vi "HAL camera program for acquisition.vi"(2 "error in":errorcluster, 3 "Camera Parameters (important)":T1={"Exposure Time (sec)"=0.0, "EM CCD Gain"=0, "Readout Settings"={"Acquisition Mode"=enum."(do not use)", "Pixel Rate"=enum."EM CCD 30 Mhz 16 bits", "High Capacity?"=FALSE, "V Shift Speed (us/row)"=enum."4.33", "V Shift Amplitude"=enum."normal", "Preamp Gain"=enum."1", "Trigger Mode"=0, "Baseline offset"=0, "Baseline clamp"=FALSE}, "Image Size"={"H Bin"=0, "V Bin"=0, "Left"=0, "Top"=0, "Right"=0, "Bottom"=0}} {"Readout Settings"."Baseline offset" min=-1000 max=1000 step=100; "Readout Settings"."Trigger Mode" items=["Internal", "External"]; "EM CCD Gain" scale=1.0..300.0; "Exposure Time (sec)" scale=0.001..10.0 scale format="%#_1g"}) -> (0 "error out":errorcluster, 1 "Actual Exposure Time (sec)":sgl)   [LabVIEW 2015]
uses:
  ixon ultra1024/HAL camera parameters important.ctt
  ixon ultra1024/ixon readout settings.ctl
  ixon ultra1024/andor acquisition mode.ctl
  Camera/camera globals.vi
panel:
  # "Camera: Andor iXon Ultra"
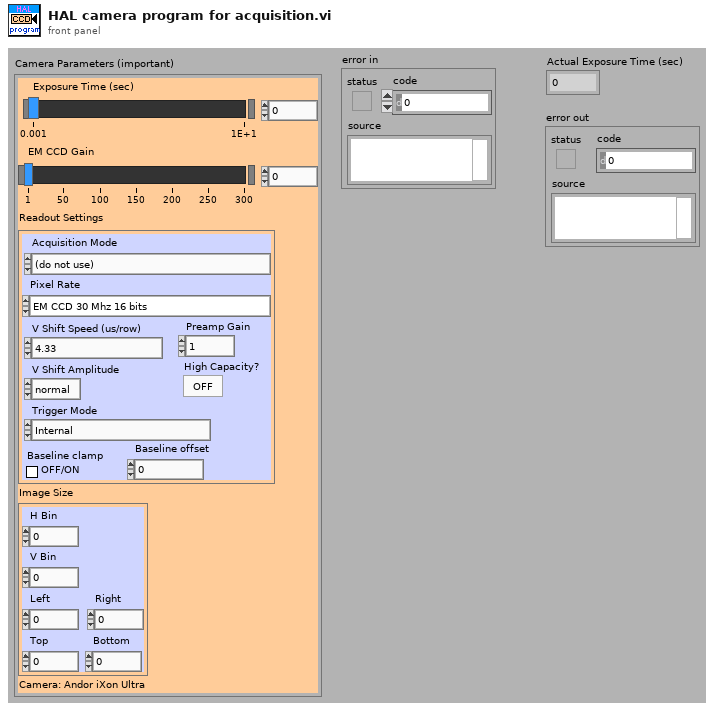
[diagram p1: front panel]
types:
  T1 = typedef "HAL camera parameters important.ctt" = cluster{"Exposure Time (sec)":sgl, "EM CCD Gain":u16, "Readout Settings":T2, "Image Size":cluster{"H Bin":i32, "V Bin":i32, "Left":i32, "Top":i32, "Right":i32, "Bottom":i32}}
  T2 = typedef "ixon readout settings.ctl" = cluster{"Acquisition Mode":T3, "Pixel Rate":enum16{"EM CCD 30 Mhz 16 bits", "EM CCD 20 Mhz 16 bits", "EM CCD 10 Mhz 16 bits", "EM CCD 1 Mhz 16 bits", "Standard CCD 1 Mhz 16 bits", "Standard CCD 0.1 Mhz 16 bits"}, "High Capacity?":bool, "V Shift Speed (us/row)":enum16{"0.6 (not reccommended)", "1.13  (not reccommended)", "2.2  (not reccommended)", "4.33"}, "V Shift Amplitude":enum16{"normal", "+1", "+2", "+3", "+4"}, "Preamp Gain":enum16{"1", "2", "3"}, "Trigger Mode":u32, "Baseline offset":i16, "Baseline clamp":bool}
  T3 = typedef "andor acquisition mode.ctl" = enum16{"(do not use)", "Single Scan", "Accumulate", "Kinetics", "Fast Kinetics", "Kinetics Run till Abort", "Frame Transfer", "Frame Transfer Run till Abort", "(do not use) ", "Time Delayed Integration"}
  T4 = cluster{"H Bin":i32, "V Bin":i32, "Left":i32, "Top":i32, "Right":i32, "Bottom":i32}
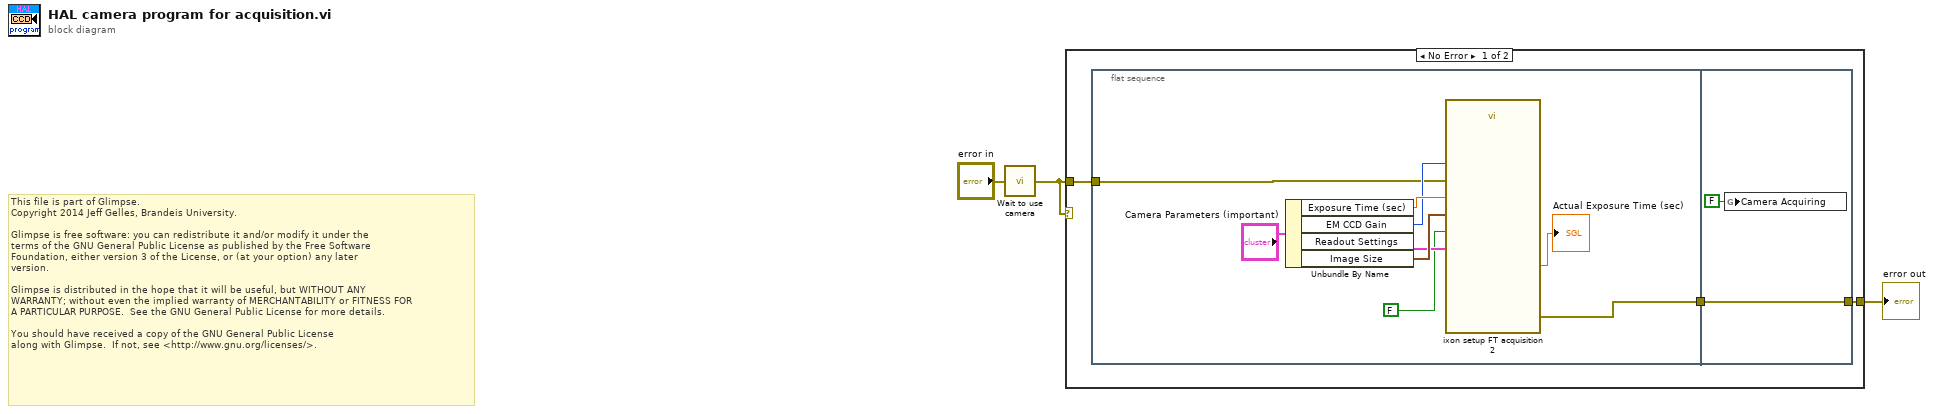
[diagram p0: block diagram]
diagram:
  # "This file is part of Glimpse. \nCopyright 2014 Jeff Gelles, Brandeis University.    \n\nGlimpse is free software: you can redistribute it and/or modify it under the \nterms of the GNU General Public License as published by the Free Software \nFoundation, either version 3 of the License, or (at your option) any later \nversion.\n\nGlimpse is distributed in the hope that it will be useful, but WITHOUT ANY \nWARRANTY; without even the implied warranty of MERCHANTABILITY or FITNESS FOR \nA PARTICULAR PURPOSE.  See the GNU General Public License for more details.\n\nYou should have received a copy of the GNU General Public License\nalong with Glimpse.  If not, see <http://www.gnu.org/licenses/>."
  n1 = call "Wait to use camera.vi"("error in"="error in") -> ("error out"=w1:errorcluster)
  n2 = case shown="No Error" w1 {
    tunnel: [w6 w18] -> w3
    tunnel: w1 -> [w5 w18]
    frame No Error {
      n3 = flat-sequence {
        tunnel: w5 -> [w7]
        tunnel: [w15] -> w4
        tunnel: [w17] -> w6
        tunnel: w4 -> [w17]
        frame #0 {
          n4 = Unbundle By Name("Camera Parameters (important)") -> ("Exposure Time (sec)"=w13:sgl, "EM CCD Gain"=w10:u16, "Readout Settings"=w11:T2, "Image Size"=w12:T4)
          n5 = call "ixon setup FT acquisition 2.vi"("EM CCD Gain"=w10, "Interactive?"=FALSE, "error in (no error)"=w7, "Exposure Time (sec)"=w13, "Readout Settings"=w11, "Image Size"=w12) -> ("error out"=w15:errorcluster, "Actual Exposure Time (sec)"=→"Actual Exposure Time (sec)":sgl)  [unwired: 1 in, 3 out]
        }
        frame #1 {
          n6 = global write "camera globals.vi" "Camera Acquiring"(FALSE ("Andor Aquiring")) -> ()
        }
      }
    }
    frame Error {
    }
  }
  "error out" <- w3
